vi "XBee_RX.vi"() -> ()   [LabVIEW 2010]
uses:
  <vilib>/Instr/_visa.llb/VISA Configure Serial Port (Instr).vi
panel:
  in  "byte count":u32=54
  out "Inverter Breaker Tripped":dbl=39.0
  out "Low Battery Voltage":dbl=39.0
  out "High Battery Voltage":dbl=39.0
  out "Heatsink Overtemp":dbl=39.0
  out "Transformer Overtemp":dbl=39.0
  out "Over Current":dbl=39.0
  out "Exercise Start Ready":dbl=39.0
  out "Voltage Start Ready":dbl=39.0
  out "Load Amp Start":dbl=39.0
  out "Generator Max Run Time Error":dbl=39.0
  out "Generator Sync Error":dbl=39.0
  out "Generator Start Error":dbl=39.0
  out "Generator Over/Under Speed Error":dbl=39.0
  out "Read Frequency Hertz":dbl=39.0
  out "Generator Volts AC":dbl=39.0
  out "Inverter Volts":dbl=39.0
  out "Temp Battery Voltage":dbl=39.0
  out "Actual Battery Voltage":dbl=39.0
  out "Load Amps":dbl=39.0
  out "Input Amps":dbl=39.0
  out "Inverter/Charger Amps AC":dbl=39.0
  out "Message Type":dbl=39.0
  in  "VISA resource name":refnum<visa-resource-name>="COM4"
  in  "stop":bool
  out "API Packet":string
  out "Active Channels":string
  out "Source Address":string="Vx"
  out "Byte Length":dbl=14.0
  out "RSSI":dbl=39.0
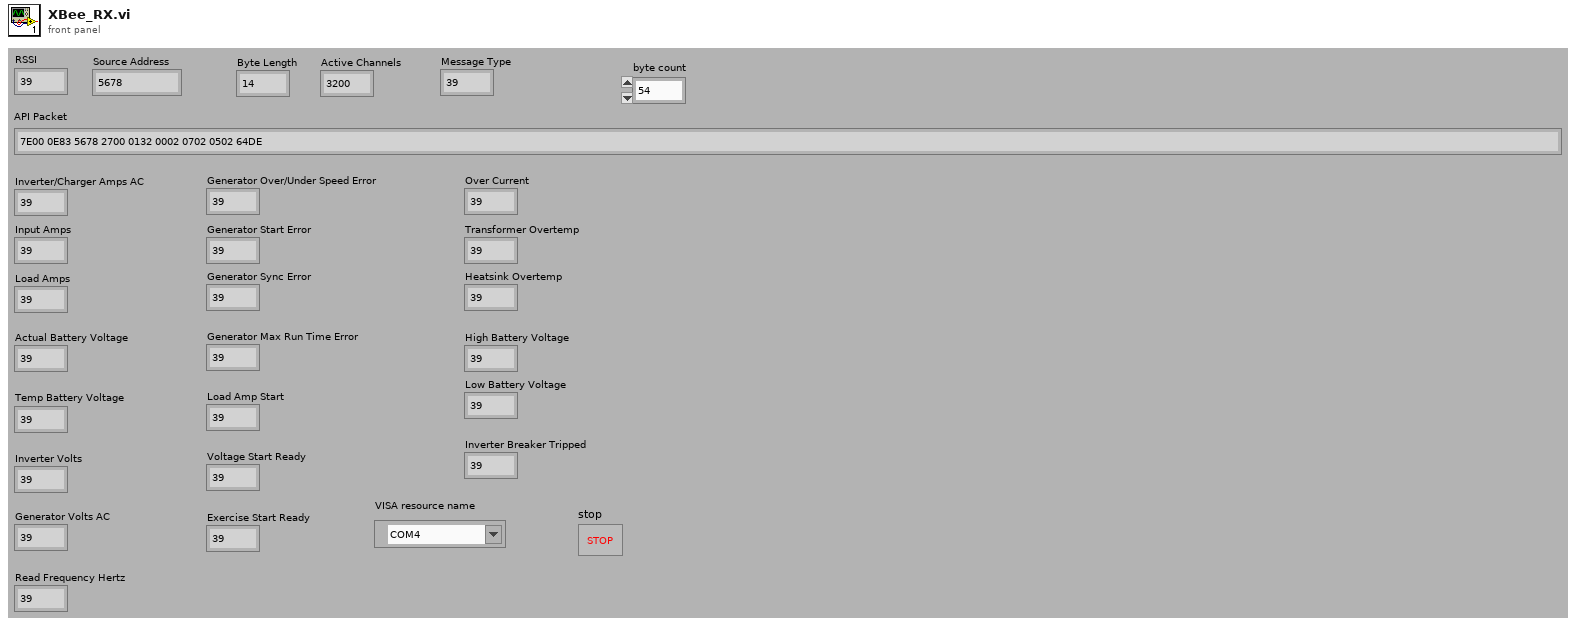
[diagram p1: front panel]
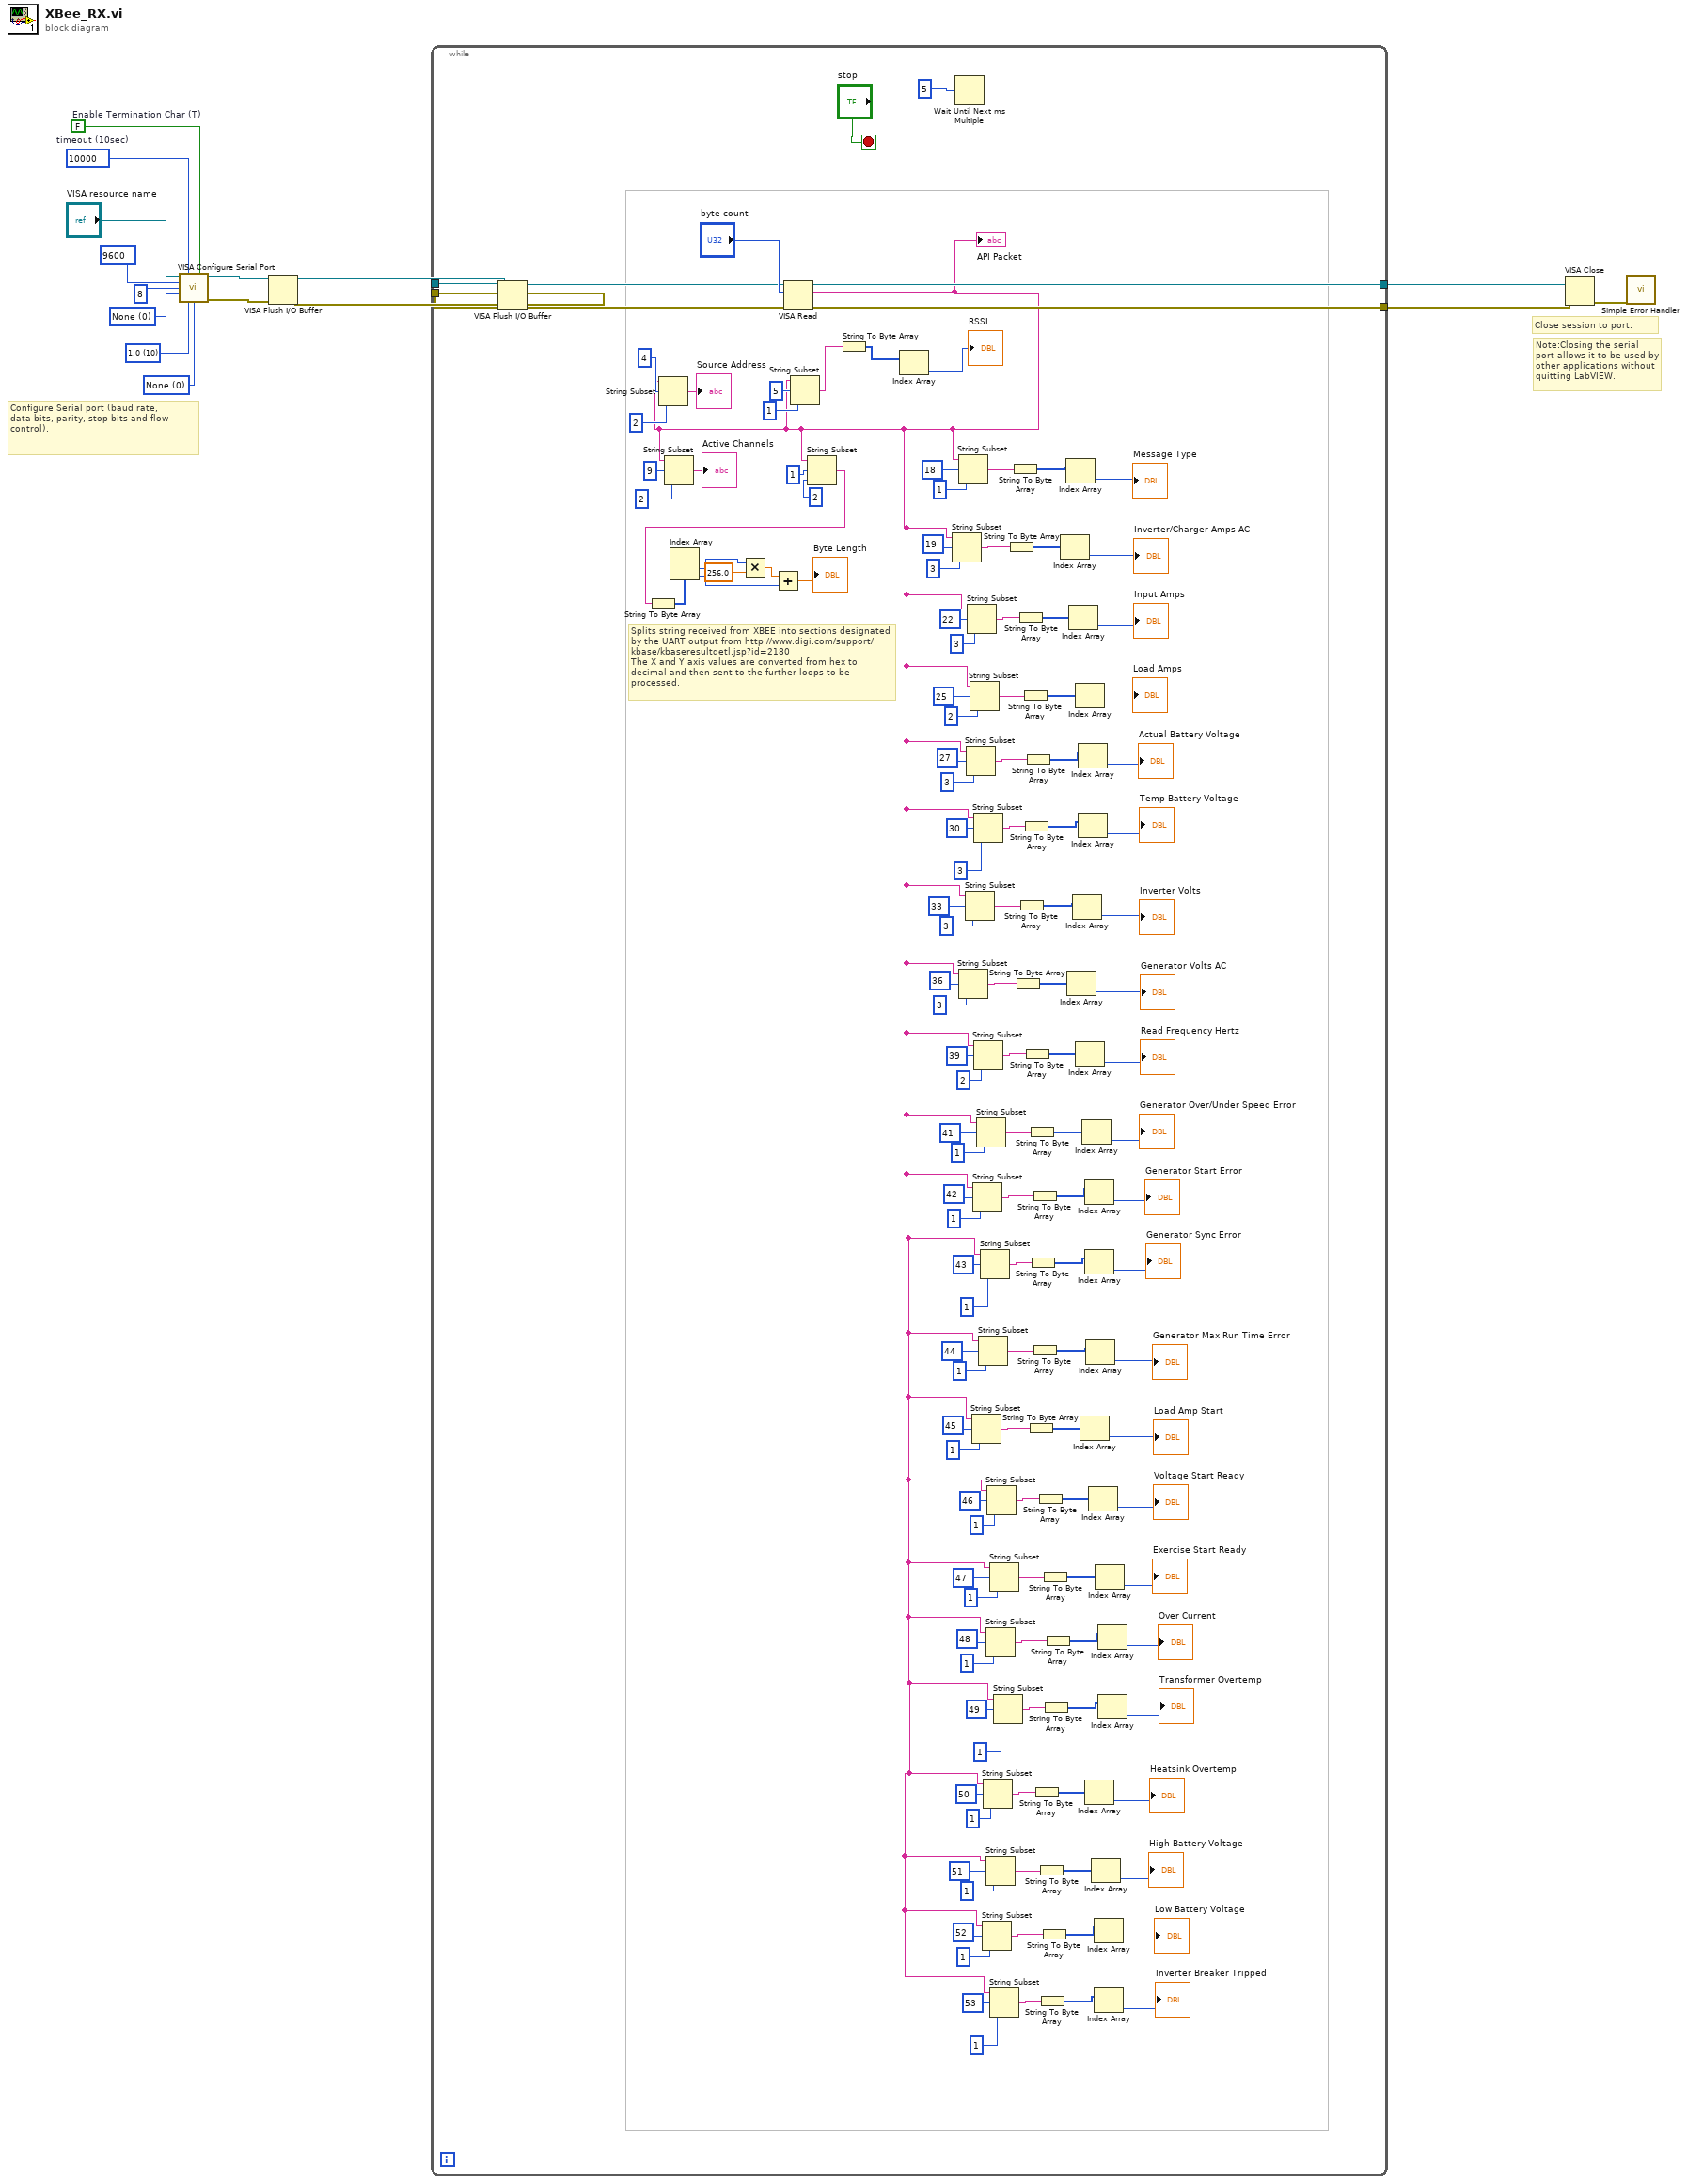
[diagram p0: block diagram]
diagram:
  w4 = u16 0 items=["None"=0, "XON/XOFF"=1, "RTS/CTS"=2, "DTR/DSR"=4] ("flow control")
  w5 = u16 10 items=["1.0"=10, "1.5"=15, "2.0"=20] ("stop bits")
  w8 = u16 0 items=["None", "Odd", "Even", "Mark", "Space"] ("parity")
  w6 = FALSE  # Enable Termination Char (T)
  w7 = u32 10000  # timeout (10sec)
  # "Configure Serial port (baud rate,\ndata bits, parity, stop bits and flow control)."
  # "Note:Closing the serial port allows it to be used by other applications without\nquitting LabVIEW."
  # "Close session to port."
  n1 = call-poly "VISA Configure Serial Port"("VISA resource name"="VISA resource name", "timeout (10sec)"=w7, "Enable Termination\nChar (T)"=w6, "baud rate (9600)"=u32 9600 ("baud rate"), "data bits (8)"=u16 8 ("data bits"), "parity (0:none)"=w8, "stop bits (10: 1 bit)"=w5, "flow control (0:none)"=w4) -> ("VISA resource name out"=w9:refnum<visa-resource-name>, "error out"=w10:errorcluster)  [unwired: 1 in, 5 out]
  n2 = VISA Flush I/O Buffer(VISA resource name=w9, error in (no error)=w10) -> (VISA resource name out=w2:refnum<visa-resource-name>, error out=w1:errorcluster)  [unwired: 1 out]
  n3 = while {
    tunnel: [w155] -> w15
    tunnel: [w154] -> w14
    tunnel: w2 -> [w18]
    tunnel: w1 -> [w19]
    stop <- "stop" stop-if-true
    # "Splits string received from XBEE into sections designated by the UART output from http://www.digi.com/support/kbase/kbaseresultdetl.jsp?id=2180 \nThe X and Y axis values are converted from hex to decimal and then sent to the further loops to be processed."
    n4 = VISA Flush I/O Buffer(VISA resource name=w18, error in (no error)=w19) -> (VISA resource name out=w17:refnum<visa-resource-name>, error out=w16:errorcluster)  [unwired: 1 out]
    n5 = VISA Read(VISA resource name=w17, byte count="byte count", error in (no error)=w16) -> (VISA resource name out=w154:refnum<visa-resource-name>, read buffer=w20:string, error out=w155:errorcluster)  [unwired: 1 out]
    "API Packet" <- w20
    n6 = String Subset(string=w20, offset (0)=4, length (rest)=2 ("length (rest)")) -> (substring=→"Source Address":string)
    n7 = String Subset(string=w20, offset (0)=9, length (rest)=2 ("length (rest)")) -> (substring=→"Active Channels":string)
    n8 = String Subset(string=w20, offset (0)=5, length (rest)=1 ("length (rest)")) -> (substring=w126:string)
    n9 = String Subset(string=w20, offset (0)=1, length (rest)=2 ("length (rest)")) -> (substring=w128:string)
    n10 = String To Byte Array(string=w128) -> (unsigned byte array=w130:u8[])
    n11 = Index Array(array=w130) -> (element #1=w133:u8, element #2=w131:u8)  [unwired: 2 in]
    n12 = Multiply(x=w133, y=256.0) -> (x*y=w132:dbl)
    n13 = Add(x=w132, y=w131) -> (x+y=→"Byte Length":dbl)
    n14 = String To Byte Array(string=w126) -> (unsigned byte array=w127:u8[])
    n15 = Index Array(array=w127) -> (element=→"RSSI":u8)  [unwired: 1 in]
    n16 = String Subset(string=w20, offset (0)=19, length (rest)=3 ("length (rest)")) -> (substring=w117:string)
    n17 = Wait Until Next ms Multiple(millisecond multiple=u32 5 ("milliseconds to wait")) -> ()  [unwired: 1 out]
    n18 = String Subset(string=w20, offset (0)=18, length (rest)=1 ("length (rest)")) -> (substring=w118:string)
    n19 = String Subset(string=w20, offset (0)=36, length (rest)=3 ("length (rest)")) -> (substring=w84:string)
    n20 = String Subset(string=w20, offset (0)=33, length (rest)=3 ("length (rest)")) -> (substring=w83:string)
    n21 = String Subset(string=w20, offset (0)=27, length (rest)=3 ("length (rest)")) -> (substring=w114:string)
    n22 = String Subset(string=w20, offset (0)=22, length (rest)=3 ("length (rest)")) -> (substring=w116:string)
    n23 = String Subset(string=w20, offset (0)=25, length (rest)=2 ("length (rest)")) -> (substring=w113:string)
    n24 = String Subset(string=w20, offset (0)=45, length (rest)=1 ("length (rest)")) -> (substring=w54:string)
    n25 = String Subset(string=w20, offset (0)=42, length (rest)=1 ("length (rest)")) -> (substring=w87:string)
    n26 = String Subset(string=w20, offset (0)=30, length (rest)=3 ("length (rest)")) -> (substring=w115:string)
    n27 = String Subset(string=w20, offset (0)=39, length (rest)=2 ("length (rest)")) -> (substring=w85:string)
    n28 = String Subset(string=w20, offset (0)=41, length (rest)=1 ("length (rest)")) -> (substring=w88:string)
    n29 = String Subset(string=w20, offset (0)=44, length (rest)=1 ("length (rest)")) -> (substring=w53:string)
    n30 = String Subset(string=w20, offset (0)=43, length (rest)=1 ("length (rest)")) -> (substring=w86:string)
    n31 = String Subset(string=w20, offset (0)=52, length (rest)=1 ("length (rest)")) -> (substring=w34:string)
    n32 = String Subset(string=w20, offset (0)=50, length (rest)=1 ("length (rest)")) -> (substring=w36:string)
    n33 = String Subset(string=w20, offset (0)=48, length (rest)=1 ("length (rest)")) -> (substring=w57:string)
    n34 = String Subset(string=w20, offset (0)=51, length (rest)=1 ("length (rest)")) -> (substring=w33:string)
    n35 = String Subset(string=w20, offset (0)=46, length (rest)=1 ("length (rest)")) -> (substring=w55:string)
    n36 = String Subset(string=w20, offset (0)=47, length (rest)=1 ("length (rest)")) -> (substring=w58:string)
    n37 = String Subset(string=w20, offset (0)=53, length (rest)=1 ("length (rest)")) -> (substring=w35:string)
    n38 = String Subset(string=w20, offset (0)=49, length (rest)=1 ("length (rest)")) -> (substring=w56:string)
    n39 = String To Byte Array(string=w117) -> (unsigned byte array=w121:u8[])
    n40 = String To Byte Array(string=w118) -> (unsigned byte array=w123:u8[])
    n41 = String To Byte Array(string=w84) -> (unsigned byte array=w80:u8[])
    n42 = String To Byte Array(string=w116) -> (unsigned byte array=w119:u8[])
    n43 = String To Byte Array(string=w83) -> (unsigned byte array=w78:u8[])
    n44 = String To Byte Array(string=w113) -> (unsigned byte array=w108:u8[])
    n45 = String To Byte Array(string=w115) -> (unsigned byte array=w112:u8[])
    n46 = String To Byte Array(string=w85) -> (unsigned byte array=w82:u8[])
    n47 = String To Byte Array(string=w114) -> (unsigned byte array=w110:u8[])
    n48 = String To Byte Array(string=w54) -> (unsigned byte array=w50:u8[])
    n49 = String To Byte Array(string=w88) -> (unsigned byte array=w93:u8[])
    n50 = String To Byte Array(string=w86) -> (unsigned byte array=w89:u8[])
    n51 = String To Byte Array(string=w87) -> (unsigned byte array=w91:u8[])
    n52 = String To Byte Array(string=w53) -> (unsigned byte array=w48:u8[])
    n53 = String To Byte Array(string=w36) -> (unsigned byte array=w37:u8[])
    n54 = String To Byte Array(string=w55) -> (unsigned byte array=w52:u8[])
    n55 = String To Byte Array(string=w33) -> (unsigned byte array=w28:u8[])
    n56 = String To Byte Array(string=w35) -> (unsigned byte array=w32:u8[])
    n57 = String To Byte Array(string=w34) -> (unsigned byte array=w30:u8[])
    n58 = String To Byte Array(string=w58) -> (unsigned byte array=w63:u8[])
    n59 = String To Byte Array(string=w56) -> (unsigned byte array=w59:u8[])
    n60 = String To Byte Array(string=w57) -> (unsigned byte array=w61:u8[])
    n61 = Index Array(array=w121) -> (element=→"Inverter/Charger Amps AC":u8)  [unwired: 1 in]
    n62 = Index Array(array=w123) -> (element=→"Message Type":u8)  [unwired: 1 in]
    n63 = Index Array(array=w80) -> (element=→"Generator Volts AC":u8)  [unwired: 1 in]
    n64 = Index Array(array=w119) -> (element=→"Input Amps":u8)  [unwired: 1 in]
    n65 = Index Array(array=w78) -> (element=→"Inverter Volts":u8)  [unwired: 1 in]
    n66 = Index Array(array=w108) -> (element=→"Load Amps":u8)  [unwired: 1 in]
    n67 = Index Array(array=w82) -> (element=→"Read Frequency Hertz":u8)  [unwired: 1 in]
    n68 = Index Array(array=w110) -> (element=→"Actual Battery Voltage":u8)  [unwired: 1 in]
    n69 = Index Array(array=w112) -> (element=→"Temp Battery Voltage":u8)  [unwired: 1 in]
    n70 = Index Array(array=w50) -> (element=→"Load Amp Start":u8)  [unwired: 1 in]
    n71 = Index Array(array=w93) -> (element=→"Generator Over/Under Speed Error":u8)  [unwired: 1 in]
    n72 = Index Array(array=w91) -> (element=→"Generator Start Error":u8)  [unwired: 1 in]
    n73 = Index Array(array=w89) -> (element=→"Generator Sync Error":u8)  [unwired: 1 in]
    n74 = Index Array(array=w37) -> (element=→"Heatsink Overtemp":u8)  [unwired: 1 in]
    n75 = Index Array(array=w48) -> (element=→"Generator Max Run Time Error":u8)  [unwired: 1 in]
    n76 = Index Array(array=w52) -> (element=→"Voltage Start Ready":u8)  [unwired: 1 in]
    n77 = Index Array(array=w28) -> (element=→"High Battery Voltage":u8)  [unwired: 1 in]
    n78 = Index Array(array=w30) -> (element=→"Low Battery Voltage":u8)  [unwired: 1 in]
    n79 = Index Array(array=w32) -> (element=→"Inverter Breaker Tripped":u8)  [unwired: 1 in]
    n80 = Index Array(array=w63) -> (element=→"Exercise Start Ready":u8)  [unwired: 1 in]
    n81 = Index Array(array=w61) -> (element=→"Over Current":u8)  [unwired: 1 in]
    n82 = Index Array(array=w59) -> (element=→"Transformer Overtemp":u8)  [unwired: 1 in]
  }
  n83 = VISA Close(VISA resource name=w14, error in (no error)=w15) -> (error out=w13:errorcluster)
  n84 = call <vilib>:"Simple Error Handler.vi"("error in (no error)"=w13) -> ()  [unwired: 1 in, 8 out]
